vi "ZMC Get Output.vi"(8 "error in (no error)":errorcluster caption="错误输入（无错误）", 9 "pistate":string, 10 "inum":u16, 11 "handle":u32) -> (0 "error out":errorcluster caption="错误输出", 1 "pistate out":string, 2 "function return":i32, 3 "handle out":u32)   [LabVIEW 2015, in "zauxdll.lvlib"]
doc: "int32 __stdcall ZMC_GetOutput(ZMC_HANDLE handle, uint16 inum, uint8* pistate);"
uses:
  zauxdll.lvlib
  zmotion.dll
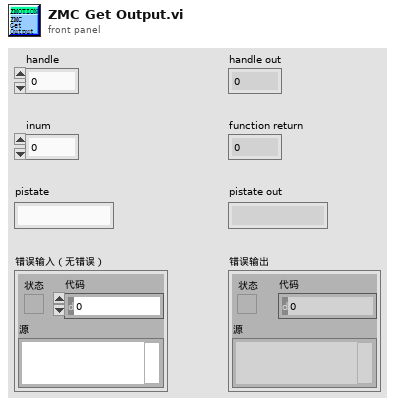
[diagram p1: front panel]
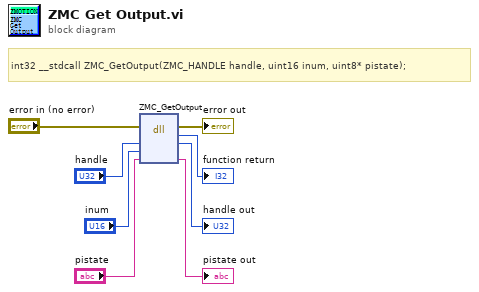
[diagram p0: block diagram]
diagram:
  # "int32 __stdcall ZMC_GetOutput(ZMC_HANDLE handle, uint16 inum, uint8* pistate);"
  n1 = dll-call lib="C:/Users/VIC/Desktop/GOGORO_SA/system/LLB/zmotion/zaux/zmotion.*" fn="ZMC_GetOutput"(error in="error in (no error)", "handle"="handle", "inum"="inum", "pistate"="pistate") -> (error out=→"error out":errorcluster, →"function return":i32, "handle"=→"handle out":u32, "pistate"=→"pistate out":string)  [unwired: 3 in, 1 out]
